vi "ConversionAndInformation.vi"() -> ()   [LabVIEW 2013]
uses:
  Unit_Control.ctl
  Constants.ctl
panel:
  in  "Tab Control":enum32{"1", "2"}(tab)
  in  "Input Type":enum16{"Frequency", "Wavelength ", "Energy"}(ring)
  in  "Input":dbl
  in  "Input Unit":T1=enum."Meter"
  out "Energy":dbl
  out "Frequency":dbl
  out "Wavelength":dbl
  in  "Output Unit 1":T1=enum."Meter"
  in  "Output Unit 2":T1=enum."Meter"
  in  "Output Unit 3":T1=enum."Meter"
  in  "Category":T2(ring)
  in  "stop":bool
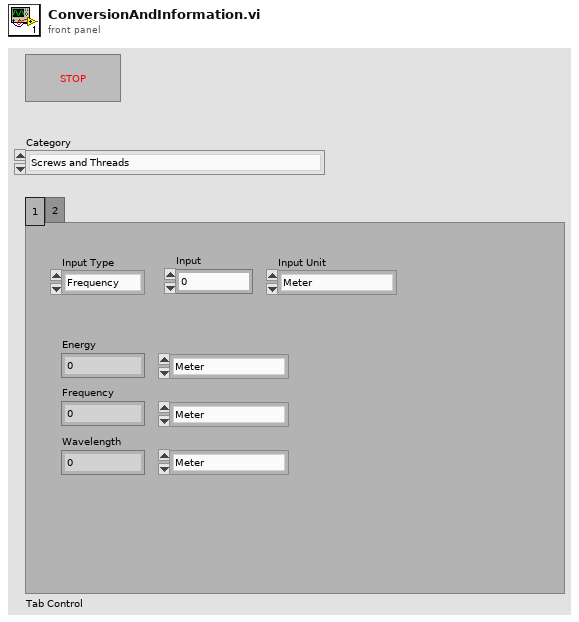
[diagram p1: front panel]
types:
  T1 = typedef "Unit_Control.ctl" = enum16{"Microsteps", "Inches", "Nanometer", "Meter", "Centimeter", "Millimeter", "Micron", "Joule", "Electron Volts", "Hertz", "Terahertz", "Megahertz"}
  T2 = enum16{"Screws and Threads", "Energy, Wavelength, Frequency"}
  T3 = typedef "Constants.ctl" = dbl
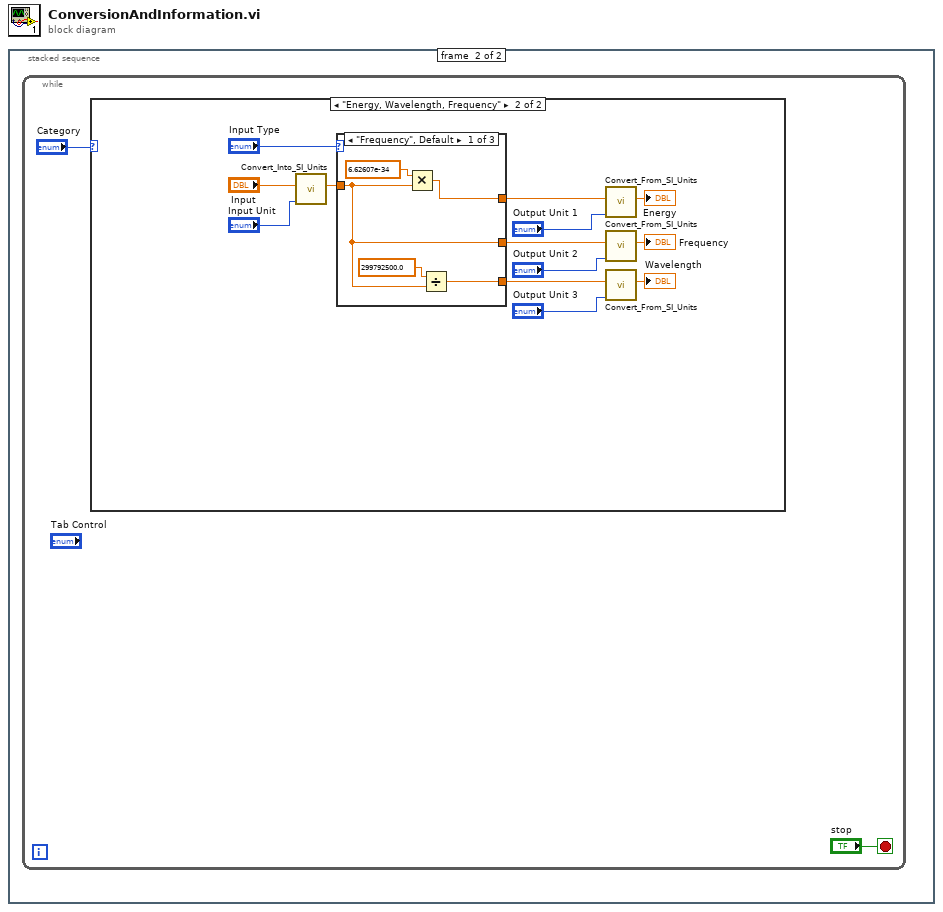
[diagram p0: block diagram]
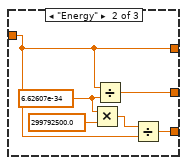
[diagram p4: hidden frame]
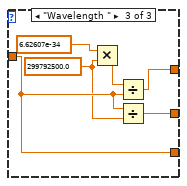
[diagram p5: hidden frame]
diagram:
  n1 = stacked-sequence {
    frame #0 {
    }
    frame #1 {
      n2 = while {
        stop <- "stop" stop-if-true
        n3 = case shown="\"Energy, Wavelength, Frequency\"" "Category" {
          frame "Screws and Threads", Default {
          }
          frame "Energy, Wavelength, Frequency" {
            n4 = call "Convert_Into_SI_Units.vi"("Input Unit"="Input Unit", "Input"="Input") -> ("Output"=w13:dbl)  [unwired: 9 in]
            n5 = case shown="\"Frequency\", Default" "Input Type" {
              tunnel: w13 -> [w19 w24 w29]
              tunnel: [w20 w24 w31] -> w11
              tunnel: [w19 w26 w30] -> w8
              tunnel: [w18 w23 w29] -> w5
              frame "Frequency", Default {
                w16 = T3 299792500.0 items=["pi (Number)"=3.141593, "e [As]"=1.602177e-19, "h [Js]"=6.62607e-34, "c [m/s]"=299792500.0, "e (Number)"=2.718282] ("Constants")
                w17 = T3 6.62607e-34 items=["pi (Number)"=3.141593, "e [As]"=1.602177e-19, "h [Js]"=6.62607e-34, "c [m/s]"=299792500.0, "e (Number)"=2.718282] ("Constants")
                n6 = Multiply(x=w17, y=w19) -> (x*y=w20:T3)
                n7 = Divide(x=w16, y=w19) -> (x/y=w18:T3)
              }
              frame "Energy" {
                w21 = T3 299792500.0 items=["pi (Number)"=3.141593, "e [As]"=1.602177e-19, "h [Js]"=6.62607e-34, "c [m/s]"=299792500.0, "e (Number)"=2.718282] ("Constants")
                w22 = T3 6.62607e-34 items=["pi (Number)"=3.141593, "e [As]"=1.602177e-19, "h [Js]"=6.62607e-34, "c [m/s]"=299792500.0, "e (Number)"=2.718282] ("Constants")
                n8 = Multiply(x=w22, y=w21) -> (x*y=w25:T3)
                n9 = Divide(x=w24, y=w22) -> (x/y=w26:T3)
                n10 = Divide(x=w25, y=w24) -> (x/y=w23:T3)
              }
              frame "Wavelength " {
                w27 = T3 6.62607e-34 items=["pi (Number)"=3.141593, "e [As]"=1.602177e-19, "h [Js]"=6.62607e-34, "c [m/s]"=299792500.0, "e (Number)"=2.718282] ("Constants")
                w28 = T3 299792500.0 items=["pi (Number)"=3.141593, "e [As]"=1.602177e-19, "h [Js]"=6.62607e-34, "c [m/s]"=299792500.0, "e (Number)"=2.718282] ("Constants")
                n11 = Multiply(x=w27, y=w28) -> (x*y=w32:T3)
                n12 = Divide(x=w32, y=w29) -> (x/y=w31:T3)
                n13 = Divide(x=w29, y=w28) -> (x/y=w30:T3)
              }
            }
            n14 = call "Convert_From_SI_Units.vi"("Output Unit"="Output Unit 1", "Input"=w11) -> ("Output"=→"Energy":dbl)  [unwired: 9 in]
            n15 = call "Convert_From_SI_Units.vi"("Output Unit"="Output Unit 2", "Input"=w8) -> ("Output"=→"Frequency":dbl)  [unwired: 9 in]
            n16 = call "Convert_From_SI_Units.vi"("Output Unit"="Output Unit 3", "Input"=w5) -> ("Output"=→"Wavelength":dbl)  [unwired: 9 in]
          }
        }
      }
    }
  }
